vi "Wait10sThenAbort.vi"() -> (0 "布尔":bool)   [LabVIEW 2018]
panel:
  in  "取消":bool
  in  "确定":bool
  # "是否重新设置量程"
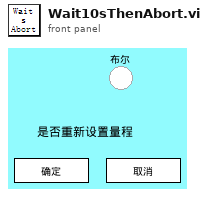
[diagram p1: front panel]
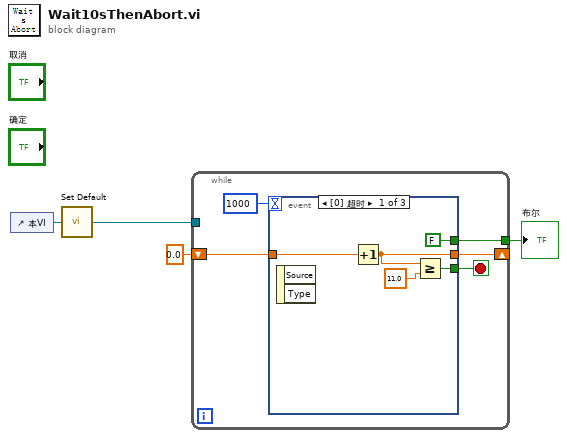
[diagram p0: block diagram]
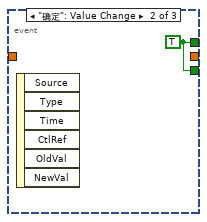
[diagram p2: hidden frame]
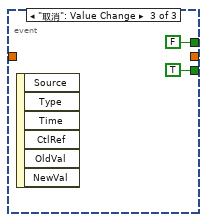
[diagram p3: hidden frame]
diagram:
  n1 = control-ref of="本VI"() -> (w2:refnum<vi>)
  n2 = call "Set Default.vi"("VI引用"=w2) -> ("引用输出"=w1:refnum<vi>)
  n3 = while {
    tunnel: [w8] -> w4
    shift-right: [w5] -> _
    shift-left: 0.0 -> [w6]
    tunnel: w1 -> [_]
    stop <- w7 stop-if-true
    n4 = event shown="[0] 超时" {
      selector: _ -> [_ _ _]
      dyn-events: _ -> [_ _ _]
      timeout: 1000 -> [_ _ _]
      tunnel: [FALSE w15 FALSE] -> w8
      tunnel: [w10 w15 TRUE] -> w7
      tunnel: w6 -> [w13 _ _]
      tunnel: [w12 _ _] -> w5
      event Timeout {
        n5 = event-data() -> ()  [unwired: 1 in, 2 out]
        n6 = Increment(x=w13) -> (x+1=w12:dbl)
        n7 = Greater Or Equal?(x=w12, y=11.0) -> (x >= y?=w10:bool)
      }
      event "确定": Value Change {
        w15 = TRUE
        n8 = event-data() -> ()  [unwired: 1 in, 6 out]
      }
      event "取消": Value Change {
        n9 = event-data() -> ()  [unwired: 1 in, 6 out]
      }
    }
  }
  "布尔" <- w4
